vi "GetBoolean.vi"(0 "Attribute":string) -> (1 "Error":bool, 2 "Boolean":bool)   [LabVIEW 2014]
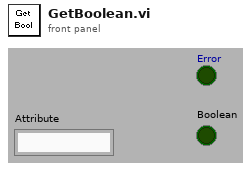
[diagram p1: front panel]
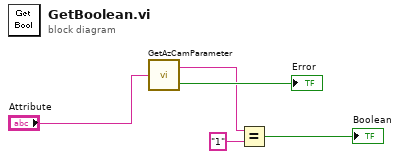
[diagram p0: block diagram]
diagram:
  n1 = call "GetAzCamParameter.vi"("Parameter"="Attribute") -> ("Error"=→"Error":bool, "Value"=w1:string)
  n2 = Equal?(x=w1, y="1") -> (x = y?=→"Boolean":bool)
